vi "GT Get Do Config.vi"(7 "pDo":T1, 8 "error in (no error)":errorcluster caption="错误输入（无错误）", 9 "doIndex":i16, 10 "doType":i16, 11 "cardNum":i16) -> (0 "error out":errorcluster caption="错误输出", 3 "function return":i16, 5 "pDo out":T1)   [LabVIEW 2020, in "gts1.lvlib"]
doc: "GT_API GT_GetDoConfig(short cardNum,short doType,short doIndex,TDoConfig *pDo);"
uses:
  gts1.lvlib
  dll/32bit/multi_card/gts.dll
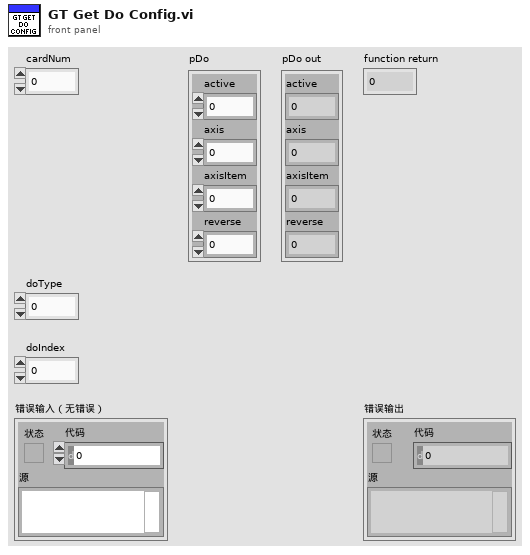
[diagram p1: front panel]
types:
  T1 = cluster{"active":i16, "axis":i16, "axisItem":i16, "reverse":i16}
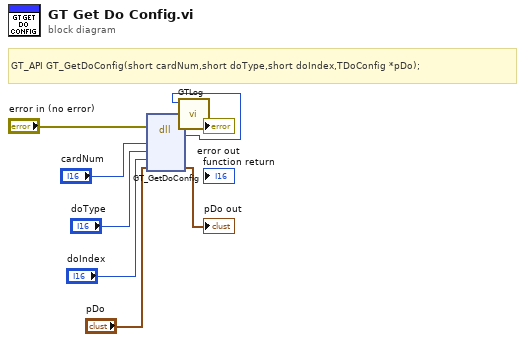
[diagram p0: block diagram]
diagram:
  # "GT_API GT_GetDoConfig(short cardNum,short doType,short doIndex,TDoConfig *pDo);"
  n1 = dll-call lib="C:/1228/dll/32bit/multi_card/gts.dll" fn="GT_GetDoConfig"(error in="error in (no error)", "cardNum"="cardNum", "doType"="doType", "doIndex"="doIndex", "pDo"="pDo") -> (error out=w3:errorcluster, w1:i16, "pDo"=→"pDo out":T1)  [unwired: 5 in, 1 out]
  n2 = call "GTLog.vi"("error in (no error)"=w3, "Numeric"=w1) -> ("error out"=→"error out":errorcluster)  [unwired: 9 in]
